vi "Main.vi"() -> ()   [LabVIEW 2021]
doc: "The Motion Sensor sample project uses the onboard accelerometer to detect motion and displays the amplitude by using the onboard LEDs of myRIO."
uses:
  <vilib>/myRIO/Instrument Drivers/Utilities/Utilities.lvlib
  <vilib>/myRIO/Express VI/Onboard Devices/LED/LED Express VI.xnode
  <vilib>/myRIO/Instrument Drivers/Onboard IO/DIO/vis/Write.vi
  <vilib>/myRIO/Instrument Drivers/Onboard IO/DIO/DIO.lvlib
  <vilib>/myRIO/Common/Instrument Driver Framework/myRIO v1.0/DIO/typedefs/DIO Channels Enum.ctl
  <vilib>/myRIO/Common/Instrument Driver Framework/myRIO v1.0/DIO/typedefs/DIO Channels List.ctl
  <vilib>/myRIO/Common/Instrument Driver Framework/Utilities/typedefs/Generic FPGA Reference.ctl
  <vilib>/myRIO/Common/Instrument Driver Framework/Utilities/typedefs/myRIO v1.0 Reference.ctl
  <vilib>/myRIO/Common/Instrument Driver Framework/Utilities/typedefs/Hardware Version Enum.ctl
  <vilib>/myRIO/Common/Instrument Driver Framework/Utilities/typedefs/myRIO Generic Hardware Reference.ctl
  <vilib>/myRIO/Instrument Drivers/Onboard IO/DIO/typedefs/DIO Reference.ctl
  <vilib>/userdefined/High Color/nirio_resource_hc.ctl
  <vilib>/myRIO/Instrument Drivers/Onboard IO/DIO/vis/myRIO DIO Open.xnode
  <vilib>/myRIO/Common/Instrument Driver Framework/Utilities/vis/Is FPGA Ref Available.vi
  <vilib>/myRIO/Express VI/Onboard Devices/Accelerometer/Accelerometer Express VI.xnode
  <vilib>/myRIO/Instrument Drivers/Onboard Devices/Accelerometer/vis/Read.vi
  <vilib>/myRIO/Instrument Drivers/Onboard Devices/Accelerometer/Accelerometer.lvlib
  <vilib>/myRIO/Common/Instrument Driver Framework/myRIO v1.0/Accelerometer/typedefs/Accelerometer Channels Enum.ctl
  <vilib>/myRIO/Common/Instrument Driver Framework/myRIO v1.0/Accelerometer/typedefs/Accelerometer Channels List.ctl
  <vilib>/myRIO/Instrument Drivers/Onboard Devices/Accelerometer/typedefs/Accelerometer Reference.ctl
  <vilib>/myRIO/Instrument Drivers/Onboard Devices/Accelerometer/vis/myRIO Accelerometer Open.xnode
  <vilib>/myRIO/Common/Instrument Driver Framework/myRIO v1.0/Accelerometer/vis/myRIO v1.1 Open Accelerometer.vi
  <vilib>/myRIO/Common/Instrument Driver Framework/myRIO v1.0/DIO/vis/myRIO v1.1 Open DIO.vi
panel:
  out "error out":errorcluster
  out "LED Status":bool[](array[boolean])
  in  "Stop":bool
  # "Overview: The Motion Sensor sample project uses the onboard accelerometer to detect motion and displays the amplitude by using the onboard LEDs of myRIO.\nInstructions:\n1. Run this VI.\n2. Shake the myRIO device."
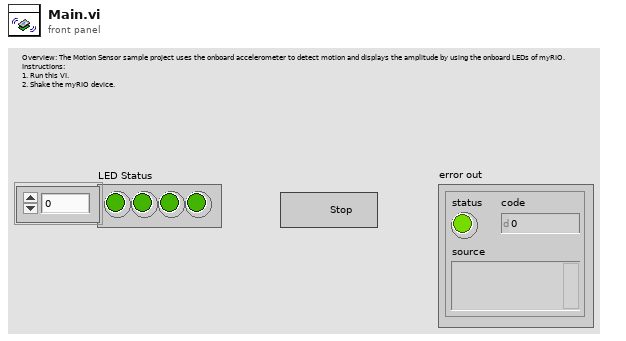
[diagram p1: front panel]
types:
  T1 = typedef "Accelerometer.lvlib/Accelerometer Reference.ctl" = cluster{"myRIO Reference":T2, "Accelerometer Channels List":T6, "LSB Weight":dbl}
  T2 = typedef "myRIO Generic Hardware Reference.ctl" = cluster{"myRIO Model":T3, "myRIO Hardware Reference":T4}
  T3 = typedef "Hardware Version Enum.ctl" = enum16{"Unknown", "myRIO-1900", "myRIO-1950", "roboRIO", "NI ELVIS RIO CM", "ELVIS III"}
  T4 = typedef "myRIO v1.0 Reference.ctl" = cluster{"Generic FPGA Reference":T5, "Allow multiple opens":bool}
  T5 = typedef "Generic FPGA Reference.ctl" = refnum<k20>
  T6 = typedef "Accelerometer Channels List.ctl" = T7[]
  T7 = typedef "Accelerometer Channels Enum.ctl" = enum16{"Not Connected", "X-Axis", "Y-Axis", "Z-Axis"}
  T8 = typedef "nirio_resource_hc.ctl" = tag
  T9 = typedef "DIO.lvlib/DIO Reference.ctl" = cluster{"myRIO Reference":T2, "DIO Channels List":T10}
  T10 = typedef "DIO Channels List.ctl" = T11[]
  T11 = typedef "DIO Channels Enum.ctl" = enum16{"Not Connected", "C/DIO0", "C/DIO1", "C/DIO2", "C/DIO3", "C/DIO4", "C/DIO5", "C/DIO6", "C/DIO7", "A/DIO0", "A/DIO1", "A/DIO2", "A/DIO3", "A/DIO4", "A/DIO5", "A/DIO6", "A/DIO7", "A/DIO8", "A/DIO9", "A/DIO10", "A/DIO11", "A/DIO12", "A/DIO13", "A/DIO14", "A/DIO15", "A/DIO16", "A/DIO17", "A/DIO18", "A/DIO19", "B/DIO0", "B/DIO1", "B/DIO2", "B/DIO3", "B/DIO4", "B/DIO5", "B/DIO6", "B/DIO7", "B/DIO8", "B/DIO9", "B/DIO10", "B/DIO11", "B/DIO12", "B/DIO13", "B/DIO14", "B/DIO15", "B/DIO16", "B/DIO17", "B/DIO18", "B/DIO19", "LED0", "LED1", "LED2", "LED3", "Button0", "DIO/DIO0", "DIO/DIO1", "DIO/DIO2", "DIO/DIO3", "DIO/DIO4", "DIO/DIO5", "DIO/DIO6", "DIO/DIO7", "DIO/DIO8", "DIO/DIO9", "SPI/CS0", "SPI/CS1", "SPI/CS2", "SPI/CS3", "LED RADIO (Green)", "LED RADIO (Red)", "LED COMM (Green)", "LED COMM (Red)", "LED MODE (Green)", "LED MODE (Red)"}
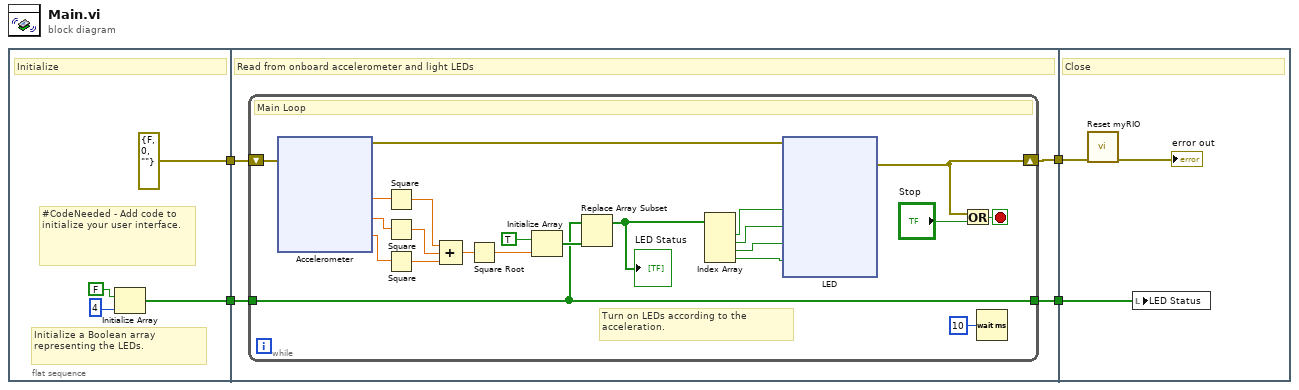
[diagram p0: block diagram]
diagram:
  n1 = flat-sequence {
    tunnel: [w6] -> w4
    tunnel: [errorcluster {"status"=FALSE, "code"=0, "source"=""} ("error out")] -> w2
    tunnel: w4 -> [w12]
    tunnel: [w11] -> w3
    tunnel: w2 -> [w10]
    tunnel: [w9] -> w1
    tunnel: w3 -> [w114]
    tunnel: w1 -> [w113]
    frame #0 {
      # "#CodeNeeded - Add code to initialize your user interface."
      # "Initialize a Boolean array representing the LEDs."
      # "Initialize"
      n2 = Initialize Array(FALSE ("element"), 4 ("dimension size")) -> (w6:bool[])
    }
    frame #1 {
      # "Read from onboard accelerometer and light LEDs"
      n3 = while {
        tunnel: w12 -> [w23]
        shift-right: [w18] -> w11
        shift-left: w10 -> [w17]
        tunnel: [w23] -> w9
        stop <- w27 stop-if-true
        # "Turn on LEDs according to the acceleration."
        # "Main Loop"
        n4 = xnode "Accelerometer"("error in (no error)"=w17) -> ("X-Axis"=w15:dbl, "Y-Axis"=w14:dbl, "Z-Axis"=w13:dbl, "error out"=w16:errorcluster)
        n5 = Square(x=w15) -> (x^2=w31:dbl)
        n6 = Square(x=w14) -> (x^2=w25:dbl)
        n7 = Square(x=w13) -> (x^2=w26:dbl)
        n8 = Compound Arithmetic op=ADD(w31, w25, w26) -> (w30:dbl)
        n9 = Square Root(x=w30) -> (sqrt(x)=w29:dbl)
        n10 = Initialize Array(TRUE ("element"), w29) -> (w33:bool[])
        n11 = Replace Array Subset(array=w23, new element=w33) -> (w32:bool[])  [unwired: 1 in]
        "LED Status" <- w32
        n12 = Index Array(array=w32) -> (element #1=w22:bool, element #2=w21:bool, element #3=w20:bool, element #4=w19:bool)  [unwired: 4 in]
        n13 = xnode "LED"("LED0"=w22, "LED1"=w21, "LED2"=w20, "LED3"=w19, "error in (no error)"=w16) -> ("error out"=w18:errorcluster)
        n14 = Or(x=w18, y="Stop") -> (x .or. y?=w27:bool)
        n15 = Wait (ms)(milliseconds to wait=u32 10) -> ()  [unwired: 1 out]
      }
    }
    frame #2 {
      # "Close"
      n16 = call <vilib>:"Reset myRIO.vi"("error in (no error)"=w114) -> ("error out"=→"error out":errorcluster)  [unwired: 10 in]
      n17 = local write "LED Status"(w113) -> ()
    }
  }
